vi "Initialize TCP_IP.vi"(8 "error in (no error)":errorcluster, 9 "Address (0)":i32, 10 "ID Query (True)":bool=TRUE, 11 "TCP/IP Address":string) -> (0 "error out":errorcluster, 3 "VISA resource name out":refnum<visa-resource-name>)   [LabVIEW 2016, in "Environment Chamber.lvlib" / "Climatic Chamber.lvlib"]
doc: "Establishes communication with the instrument and optionally performs an instrument identification query.\nTherefore, call this VI before calling other instrument driver VIs for this instrument.\nGenerally, you need to call the Initialize VI only once at the beginning of an application.\n\n<b>TCP/IP Communication</b>"
uses:
  Climatic Chamber.lvlib
panel:
  # "(c) 2015 <Espec Corp.>.  ALL RIGHTS RESERVED."
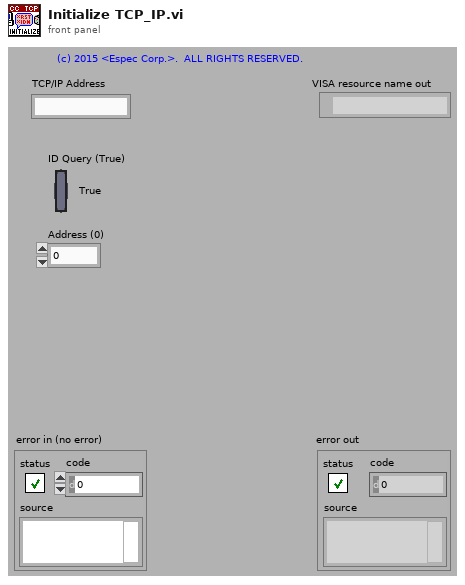
[diagram p1: front panel]
types:
  T1 = typedef "Environment Chamber.lvlib/Climatic Chamber.lvlib/Chamber Type Cluster.ctl" = cluster{"dry bulb sensor":T2, "Temp. only chamber":bool, "wet bulb sensor":T2, "Controller type":string, "Temp. upper limit":dbl}
  T2 = typedef "Environment Chamber.lvlib/Climatic Chamber.lvlib/Sensor Type Enum.ctl" = enum16{"Not defined", "Thermocouple"}
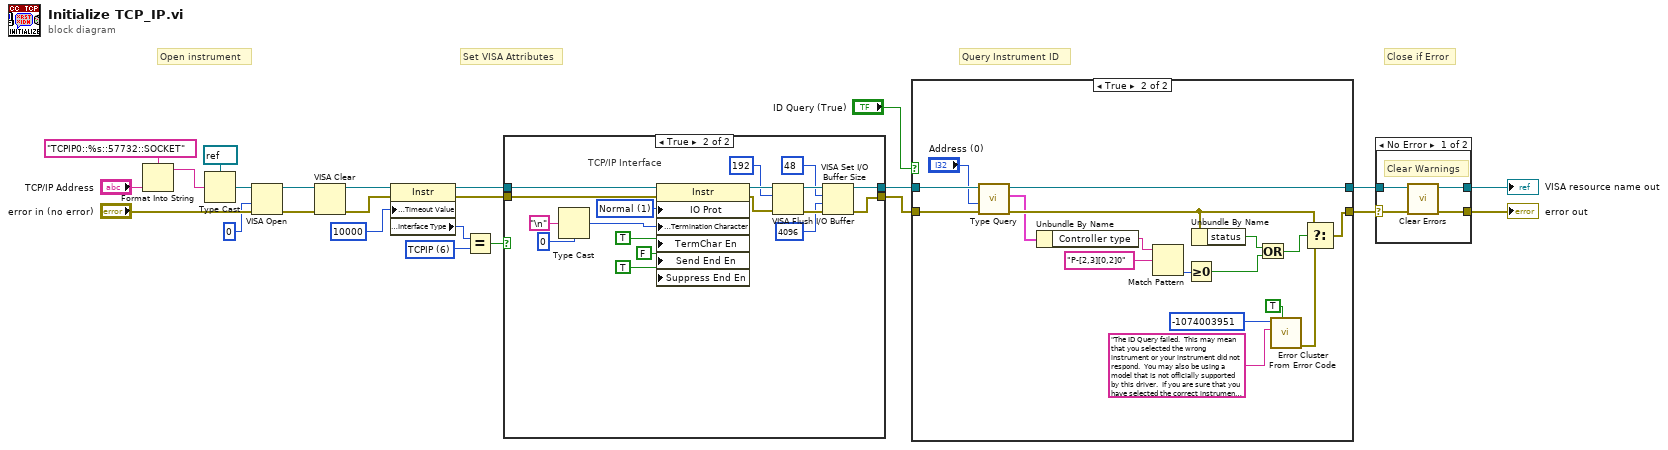
[diagram p0: block diagram]
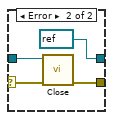
[diagram p3: hidden frame]
diagram:
  w15 = u16 6 items=["GPIB"=1, "VXI"=2, "GPIB-VXI"=3, "Serial"=4, "PXI"=5, "TCPIP"=6, "USB"=7] ("Interface Information:Interface Type")
  # "Set VISA Attributes"
  # "Close if Error"
  # "Query Instrument ID"
  # "Open instrument"
  n1 = Format Into String(format string="TCPIP0::%s::57732::SOCKET", "TCP/IP Address") -> (resulting string=w3:string)  [unwired: 2 in, 1 out]
  n2 = Type Cast(type=refnum<visa-resource-name> refnum ("VISA resource name"), x=w3) -> (*(type *) &x=w2:refnum<visa-resource-name>)
  n3 = VISA Open(access mode=u32 0, error in (no error)="error in (no error)", VISA resource name=w2) -> (VISA resource name=w13:refnum<visa-resource-name>, error out=w12:errorcluster)  [unwired: 2 in]
  n4 = VISA Clear(VISA resource name=w13, error in (no error)=w12) -> (VISA resource name out=w11:refnum<visa-resource-name>, error out=w10:errorcluster)
  n5 = property class="Instr"(reference=w11, error in=w10, "General Settings:Timeout Value"=u32 10000) -> (reference out=w18:refnum<visa-resource-name>, error out=w17:errorcluster, "Interface Information:Interface Type"=w22:u16)
  n6 = Equal?(x=w22, y=w15) -> (x = y?=w16:bool)
  n7 = case shown="True" w16 {
    tunnel: [w25 w41] -> w20
    tunnel: [w26 w38] -> w19
    tunnel: w18 -> [w25 w43]
    tunnel: w17 -> [w26 w44]
    frame False {
      # "EDIT: Remove interfaces not\nsupported by your instrument."
      # "GPIB, Serial, and USB Interface"
    }
    frame True {
      w30 = u16 1 items=["Normal"=1, "VXI/FDC"=2, "GPIB/HS488"=3, "Serial-TCPIP-USB/488 Strings"=4, "USBTMC/Vendor-Specific"=5] ("Message Based Settings:IO Protocol")
      # "TCP/IP Interface"
      n8 = Type Cast(type=u8 0, x="\n" ("Line Feed Constant")) -> (*(type *) &x=w31:u8)
      n9 = property class="Instr"(reference=w43, error in=w44, "IO Prot"=w30, "Message Based Settings:Termination Character"=w31, "TermChar En"=TRUE ("Message Based Settings:Send End Enable"), "Send End En"=FALSE ("Message Based Settings:Send End Enable"), "Suppress End En"=TRUE ("Message Based Settings:Suppress End Enable")) -> (reference out=w37:refnum<visa-resource-name>, error out=w40:errorcluster)
      n10 = VISA Flush I/O Buffer(VISA resource name=w37, mask (16)=u16 192, error in (no error)=w40) -> (VISA resource name out=w42:refnum<visa-resource-name>, error out=w39:errorcluster)
      n11 = VISA Set I/O Buffer Size(VISA resource name=w42, mask (16)=u16 48, size (4096)=u32 4096 ("size (0)"), error in (no error)=w39) -> (VISA resource name out=w41:refnum<visa-resource-name>, error out=w38:errorcluster)
    }
  }
  n12 = case shown="True" "ID Query (True)" {
    tunnel: [w45 w63] -> w6
    tunnel: [w46 w50] -> w7
    tunnel: w20 -> [w46 w51]
    tunnel: w19 -> [w45 w53]
    frame False {
    }
    frame True {
      n13 = call "Type Query.vi"("error in (no error)"=w53, "Address (0)"="Address (0)", "VISA resource name"=w51) -> ("error out"=w52:errorcluster, "Chamber Type"=w48:T1, "VISA resource name out"=w50:refnum<visa-resource-name>)  [unwired: 6 in]
      n14 = Unbundle By Name(w48) -> ("Controller type"=w47:string)
      n15 = Match Pattern(string=w47, regular expression="P-[2,3][0,2]0") -> (offset past match=w57:i32)  [unwired: 1 in, 3 out]
      n16 = Greater Or Equal To 0?(x=w57) -> (x >= 0?=w55:bool)
      n17 = Unbundle By Name(w52) -> ("status"=w56:bool)
      n18 = Or(x=w56, y=w55) -> (x .or. y?=w54:bool)
      n19 = call <vilib>:"Error Cluster From Error Code.vi"("show call chain? (False)"=TRUE, "error message (\"\")"="The ID Query failed.  This may mean that you selected the wrong instrument or your instrument did not respond.  You may also be using a model that is not officially supported by this driver.  If you are sure that you have selected the correct instrument and it is responding, try disabling the ID Query." ("Source (VI Name)"), "error code (0)"=-1074003951 ("Code")) -> ("error out"=w61:errorcluster)  [unwired: 6 in]
      n20 = Select(t=w52, s=w54, f=w61) -> (s? t:f=w63:errorcluster)
    }
  }
  n21 = case shown="No Error" w6 {
    selector: w6 -> [w65 w68]
    tunnel: w7 -> [w66 w69]
    tunnel: [w66 refnum<visa-resource-name> refnum ("VISA resource name out")] -> w9
    tunnel: [w64 w70] -> w8
    frame No Error {
      # "Clear Warnings"
      n22 = call <vilib>:"Clear Errors.vi"("error in (no error)"=w65) -> ("error out"=w64:errorcluster)  [unwired: 5 in, 1 out]
    }
    frame Error {
      n23 = call "Close.vi"("error in (no error)"=w68, "VISA resource name"=w69) -> ("error out"=w70:errorcluster)  [unwired: 9 in]
    }
  }
  "VISA resource name out" <- w9
  "error out" <- w8
